vi "rvc Interpolate Matrix Transformation.vi"(7 "ratio":dbl, 10 "final transformation":T1, 11 "initial transformation":T1) -> (3 "interpolated matrix":T1)   [LabVIEW 2013]
uses:
  <vilib>/Analysis/Matrix/Datatypes/RealMatrix.ctl
  <vilib>/Analysis/baseanly.llb/Dot Product.vi
  <vilib>/Analysis/baseanly.llb/Real Dot Product.vi
  <vilib>/Analysis/baseanly.llb/Outer Product.vi
  <vilib>/Analysis/baseanly.llb/Real Outer Product.vi
  <vilib>/robotics/Kinematics/Create Lie Group Matrix.vi
  <vilib>/robotics/Kinematics/Rotation Matrix to Angle Vector.vi
  <vilib>/Analysis/Matrix/Numeric/Multiply/Multiply.vi
  <vilib>/Analysis/Matrix/Numeric/Multiply/Multiply - RM,R.vi
  <vilib>/Analysis/Matrix/Numeric/Multiply/Multiply - R,RM.vi
  <vilib>/Analysis/Matrix/Numeric/Add/Add.vi
  <vilib>/Analysis/Matrix/Numeric/Add/Add - RM,RM.vi
  <vilib>/robotics/Kinematics/NI_Kinematics.lvlib
  <vilib>/Analysis/Matrix/NI_Matrix.lvlib
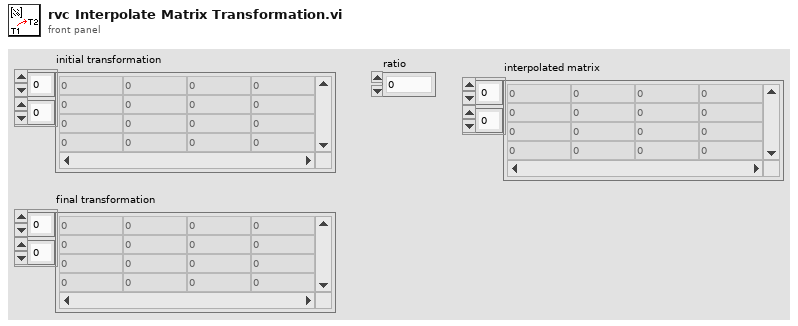
[diagram p1: front panel]
types:
  T1 = typedef "NI_Matrix.lvlib/RealMatrix.ctl" = dbl[][]
  T2 = typedef "NI_Kinematics.lvlib/Quaternion.ctl" = dbl[]
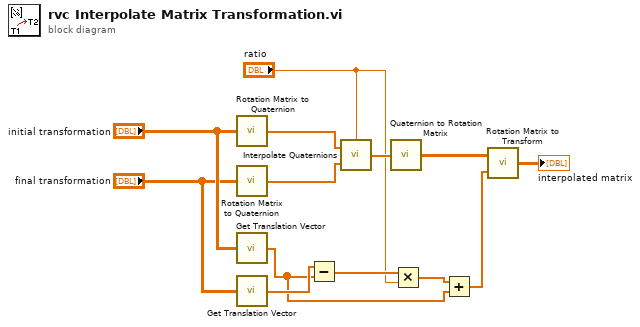
[diagram p0: block diagram]
diagram:
  n1 = call <vilib>:"Rotation Matrix to Quaternion.vi"("rotation matrix"="initial transformation") -> ("quaternion"=w12:T2)
  n2 = call <vilib>:"Rotation Matrix to Quaternion.vi"("rotation matrix"="final transformation") -> ("quaternion"=w13:T2)
  n3 = call <vilib>:"Get Translation Vector.vi"("transform"="initial transformation") -> ("translation vector"=w4:dbl[])
  n4 = call <vilib>:"Get Translation Vector.vi"("transform"="final transformation") -> ("translation vector"=w8:dbl[])
  n5 = Subtract(x=w8, y=w4) -> (x-y=w7:dbl[])
  n6 = call <vilib>:"Interpolate Quaternions.vi"("ratio"="ratio", "quaternion 2"=w13, "quaternion 1"=w12) -> ("interpolated quaternion"=w11:T2)
  n7 = call <vilib>:"Quaternion to Rotation Matrix.vi"("quaternion"=w11) -> ("rotation matrix"=w3:T1)
  n8 = Multiply(x=w7, y="ratio") -> (x*y=w5:dbl[])
  n9 = Add(x=w5, y=w4) -> (x+y=w1:dbl[])
  n10 = call <vilib>:"Rotation Matrix to Transform.vi"("translation vector"=w1, "rotation matrix"=w3) -> ("transform"=→"interpolated matrix":T1)
